vi "FGV_DO_Task.vi"(3 "error in":errorcluster, 4 "task out 2":refnum<k21> caption="DO_task", 5 "Action":T1) -> (0 "error out":errorcluster, 1 "CO task":refnum<k21> caption="DO task")   [LabVIEW 2025]
uses:
  Controls/TypeDef_FGV.ctl
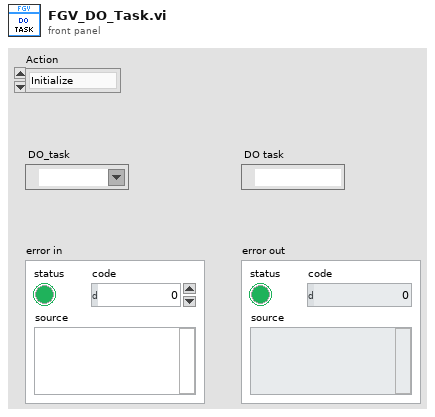
[diagram p1: front panel]
types:
  T1 = typedef "TypeDef_FGV.ctl" = enum16{"Initialize", "Write", "Read"}
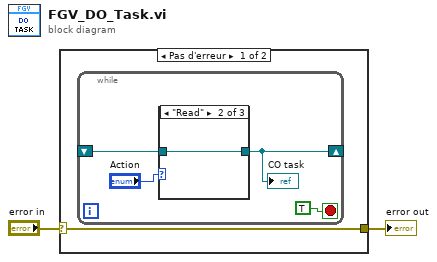
[diagram p0: block diagram]
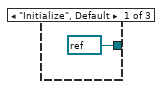
[diagram p2: hidden frame]
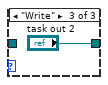
[diagram p3: hidden frame]
diagram:
  n1 = case shown="Pas d'erreur" "error in" {
    selector: "error in" -> [w3 w11]
    tunnel: [w3 w11] -> w2
    frame No Error {
      n2 = while {
        shift-right: [w4] -> _
        shift-left: _ -> [w5]
        stop <- TRUE stop-if-true
        n3 = case shown="\"Read\"" "Action" {
          tunnel: w5 -> [_ w9 _]
          tunnel: [refnum<k21> refnum ("task out") w9 "task out 2"] -> w4
          frame "Initialize", Default {
          }
          frame "Read" {
          }
          frame "Write" {
          }
        }
        "CO task" <- w4
      }
    }
    frame Error {
    }
  }
  "error out" <- w2
